vi "Get Calibration Status.vi"(8 "error in (no error)":errorcluster, 11 "BNO055 in":refnum<class "BNO055.lvclass">) -> (0 "error out":errorcluster, 2 "Calibration Status":T1, 3 "BNO055 out":refnum<class "BNO055.lvclass">)   [LabVIEW 2020, in "BNO055.lvlib" / "BNO055.lvclass"]
uses:
  BNO055.lvclass
  Calibration Status.ctl
  Paged Register.ctl
  BNO055.lvclass/BNO055.ctl
  <vilib>/MakerHub/LINX/Private/Local IO/LinxI2cWrite.vi
  <vilib>/MakerHub/LINX/Public/Utilities/Check Channel.vi
  <vilib>/MakerHub/LINX/Private/Local IO/Handle Errors.vi
  <vilib>/MakerHub/LINX/Private/Utilties/Generate Error.vi
  <vilib>/MakerHub/LINX/LMH-LINX.lvlib
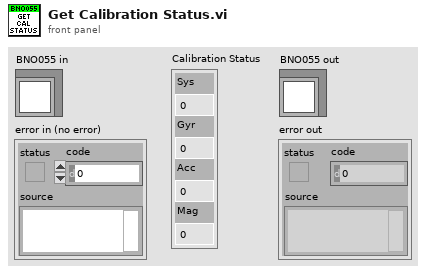
[diagram p1: front panel]
types:
  T1 = typedef "BNO055.lvlib/BNO055.lvclass/Calibration Status.ctl" = cluster{"Sys":u8, "Gyr":u8, "Acc":u8, "Mag":u8}
  T2 = typedef "BNO055.lvlib/BNO055.lvclass/Paged Register.ctl" = u16
  T3 = typedef "LMH-LINX.lvlib/LINX Ref.ctl" = cluster{"IO":T4, "Interface":T5, "LINX Device Config":T6}
  T4 = typedef "LMH-LINX.lvlib/Platform.ctl" = enum16{"Remote", "Local"}
  T5 = typedef "LMH-LINX.lvlib/Interface.ctl" = enum16{"Serial", "TCP"}
  T6 = typedef "LMH-LINX.lvlib/Device.lvlib/LINX Device Config.ctl" = cluster{"Interface":T5, "COM Port":refnum<visa-resource-name>, "TCP Configuration":T7, "Device Family":u8, "Device ID":u8, "Device Name":string, "TCP Ref":refnum<k5>, "Channels":T8}
  T7 = typedef "LMH-LINX.lvlib/Device.lvlib/TCP Config.ctl" = cluster{"IP Address":string, "Port":u16}
  T8 = typedef "LMH-LINX.lvlib/Channels.ctl" = cluster{"DI":u8[], "DO":u8[], "AI":u8[], "AO":u8[], "PWM":u8[], "QE":u8[], "UART":u8[], "I2C 2":u8[], "SPI":u8[], "CAN":u8[], "Servo":u8[], "AI Ref (V)":dbl, "AI Resolution (Bits)":u8, "AO Ref (V)":dbl, "AO Resolution (Bits)":u8}
  T9 = typedef "BNO055.lvlib/BNO055.lvclass/Address.ctl" = u8
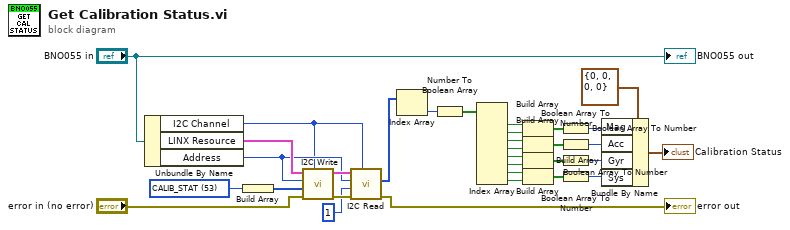
[diagram p0: block diagram]
diagram:
  w26 = T2 53 items=["CHIP_ID"=0, "ACC_ID"=1, "MAG_ID"=2, "GYR_ID"=3, "SW_REV_ID_LSB"=4, "SW_REV_ID_MSB"=5, "BL_Rev_ID"=6, "Page ID (Page 0)"=7, "ACC_DATA_X_LSB"=8, "ACC_DATA_X_MSB"=9, "ACC_DATA_Y_LSB"=10, "ACC_DATA_Y_MSB"=11, "ACC_DATA_Z_LSB"=12, "ACC_DATA_Z_MSB"=13, "MAG_DATA_X_LSB"=14, "MAG_DATA_X_MSB"=15, "MAG_DATA_Y_LSB"=16, "MAG_DATA_Y_MSB"=17, "MAG_DATA_Z_LSB"=18, "MAG_DATA_Z_MSB"=19, "GYR_DATA_X_LSB"=20, "GYR_DATA_X_MSB"=21, "GYR_DATA_Y_LSB"=22, "GYR_DATA_Y_MSB"=23, "GYR_DATA_Z_LSB"=24, "GYR_DATA_Z_MSB"=25, "EUL_Heading_LSB"=26, "EUL_Heading_MSB"=27, "EUL_Roll_LSB"=28, "EUL_Roll_MSB"=29, "EUL_Pitch_LSB"=30, "EUL_Pitch_MSB"=31, "QUA_Data_w_LSB"=32, "QUA_Data_w_MSB"=33, "QUA_Data_x_LSB"=34, "QUA_Data_x_MSB"=35, "QUA_Data_y_LSB"=36, "QUA_Data_y_MSB"=37, "QUA_Data_z_LSB"=38, "QUA_Data_z_MSB"=39, "LIA_Data_X_LSB"=40, "LIA_Data_X_MSB"=41, "LIA_Data_Y_LSB"=42, "LIA_Data_Y_MSB"=43, "LIA_Data_Z_LSB"=44, "LIA_Data_Z_MSB"=45, "GRV_Data_X_LSB"=46, "GRV_Data_X_MSB"=47, "GRV_Data_Y_LSB"=48, "GRV_Data_Y_MSB"=49, "GRV_Data_Z_LSB"=50, "GRV_Data_Z_MSB"=51, "TEMP"=52, "CALIB_STAT"=53, "ST_RESULT"=54, "INT_STA"=55, "SYS_CLK_STATUS"=56, "SYS_STATUS"=57, "SYS_ERR"=58, "UNIT_SEL"=59, "OPR_MODE"=61, "PWR_MODE"=62, "SYS_TRIGGER"=63, "TEMP_SOURCE"=64, "AXIS_MAP_CONFIG"=65, "AXIS_MAP_SIGN"=66, "ACC_OFFSET_X_LSB"=85, "ACC_OFFSET_X_MSB"=86, "ACC_OFFSET_Y_LSB"=87, "ACC_OFFSET_Y_MSB"=88, "ACC_OFFSET_Z_LSB"=89, "ACC_OFFSET_Z_MSB"=90, "MAG_OFFSET_X_LSB"=91, "MAG_OFFSET_X_MSB"=92, "MAG_OFFSET_Y_LSB"=93, "MAG_OFFSET_Y_MSB"=94, "MAG_OFFSET_Z_LSB"=95, "MAG_OFFSET_Z_MSB"=96, "GYR_OFFSET_X_LSB"=97, "GYR_OFFSET_X_MSB"=98, "GYR_OFFSET_Y_LSB"=99, "GYR_OFFSET_Y_MSB"=100, "GYR_OFFSET_Z_LSB"=101, "GYR_OFFSET_Z_MSB"=102, "ACC_RADIUS_LSB"=103, "ACC_RADIUS_MSB"=104, "MAG_RADIUS_LSB"=105, "MAG_RADIUS_MSB"=106, "Page ID (Page 1)"=263, "ACC_Config"=264, "MAG_Config"=265, "GYR_Config_0"=266, "GYR_Config_1"=267, "ACC_Sleep_Config"=268, "GYR_Sleep_Config"=269, "INT_MASK"=271, "INT_EN"=272, "ACC_AM_THRES"=273, "ACC_INT_Settings"=274, "ACC_HG_DURATION"=275, "ACC_HG_THRES"=276, "ACC_NM_THRE"=277, "ACC_NM_SET"=278, "GYR_INT_SETTING"=279, "GYR_HR_X_SET"=280, "GYR_DUR_X"=281, "GYR_HR_Y_SET"=282, "GYR_DUR_Y"=283, "GYR_HR_Z_SET"=284, "GYR_DUR_Z"=285, "GYR_AM_THRES"=286, "GYR_AM_SET"=287, "UNIQUE_ID_0"=336, "UNIQUE_ID_1"=337, "UNIQUE_ID_2"=338, "UNIQUE_ID_3"=339, "UNIQUE_ID_4"=340, "UNIQUE_ID_5"=341, "UNIQUE_ID_6"=342, "UNIQUE_ID_7"=343, "UNIQUE_ID_8"=344, "UNIQUE_ID_9"=345, "UNIQUE_ID_10"=346, "UNIQUE_ID_11"=347, "UNIQUE_ID_12"=348, "UNIQUE_ID_13"=349, "UNIQUE_ID_14"=350, "UNIQUE_ID_15"=351] ("Paged Register")
  n1 = Unbundle By Name("BNO055 in") -> ("I2C Channel"=w3:u8, "LINX Resource"=w30:T3, "Address"=w28:T9)
  n2 = Build Array(w26) -> (w25:T2[])
  n3 = call <vilib>:"I2C Write.vi"("I2C Channel"=w3, "Error In"="error in (no error)", "Data"=w25, "I2C Slave Address (0)"=w28, "LINX Resource"=w30) -> ("Error Out"=w32:errorcluster, "LINX Resource"=w29:T3)  [unwired: 5 in]
  n4 = call <vilib>:"I2C Read.vi"("I2C Channel"=w3, "Error In"=w32, "Bytes To Read"=u8 1, "I2C Slave Address (0)"=w28, "LINX Resource"=w29) -> ("Error Out"=→"error out":errorcluster, "Data"=w24:u8[])  [unwired: 4 in, 1 out]
  n5 = Index Array(array=w24) -> (element=w23:u8)  [unwired: 1 in]
  n6 = Number To Boolean Array(number=w23) -> (Boolean array=w22:bool[])
  n7 = Index Array(array=w22) -> (element #1=w21:bool, element #2=w20:bool, element #3=w19:bool, element #4=w18:bool, element #5=w17:bool, element #6=w16:bool, element #7=w15:bool, element #8=w14:bool)  [unwired: 8 in]
  n8 = Build Array(w21, w20) -> (w13:bool[])
  n9 = Build Array(w19, w18) -> (w12:bool[])
  n10 = Build Array(w17, w16) -> (w11:bool[])
  n11 = Build Array(w15, w14) -> (w10:bool[])
  n12 = Boolean Array To Number(Boolean array=w13) -> (number=w7:u32)
  n13 = Boolean Array To Number(Boolean array=w12) -> (number=w6:u32)
  n14 = Boolean Array To Number(Boolean array=w11) -> (number=w5:u32)
  n15 = Boolean Array To Number(Boolean array=w10) -> (number=w4:u32)
  n16 = Bundle By Name(cluster=T1 {"Sys"=0, "Gyr"=0, "Acc"=0, "Mag"=0} ("Calibration Status"), "Mag"=w7, "Acc"=w6, "Gyr"=w5, "Sys"=w4) -> (→"Calibration Status":T1)
  "BNO055 out" <- "BNO055 in"
